vi "Move.vi"(8 "error in (no error)":errorcluster, 11 "Snake in":refnum<class "SnakeGame.lvclass">) -> (0 "error out":errorcluster, 3 "Snake out":refnum<class "SnakeGame.lvclass">)   [LabVIEW 2019, in "RT_Game.lvlib" / "SnakeGame.lvclass"]
uses:
  SnakeGame.lvclass
  SnakeGame.lvclass/SnakeGame.ctl
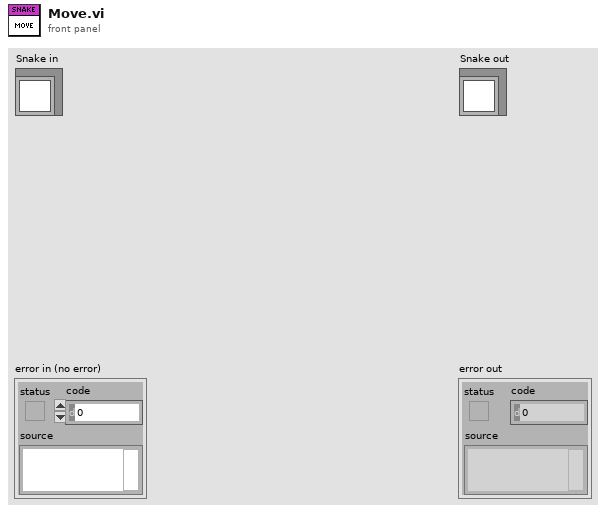
[diagram p1: front panel]
types:
  T1 = typedef "RT_Game.lvlib/SnakeGame.lvclass/Direction.ctl" = enum16{"Up", "Left", "Down", "Right"}
  T2 = typedef "RT_Game.lvlib/Game.lvclass/Coordinate.ctl" = cluster{"x":i16, "y":i16}
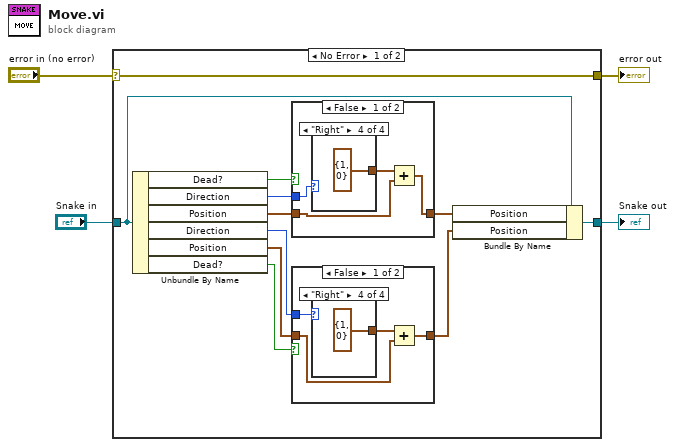
[diagram p0: block diagram]
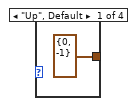
[diagram p2: hidden frame]
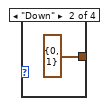
[diagram p3: hidden frame]
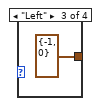
[diagram p4: hidden frame]
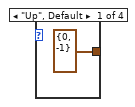
[diagram p6: hidden frame]
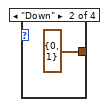
[diagram p7: hidden frame]
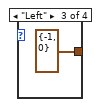
[diagram p8: hidden frame]
diagram:
  n1 = case shown="No Error" "error in (no error)" {
    selector: "error in (no error)" -> [w15 w35]
    tunnel: [w15 w35] -> w3
    tunnel: [w12 w34] -> w1
    tunnel: "Snake in" -> [w14 w34]
    frame No Error {
      n2 = Unbundle By Name(w14) -> ("Dead?"=w5:bool, "Direction"=w13:T1, "Position"=w11:T2, "Direction"=w8:T1, "Position"=w9:T2, "Dead?"=w6:bool)
      n3 = case shown="False" w5 {
        tunnel: w13 -> [w19 _]
        tunnel: w11 -> [w18 w24]
        tunnel: [w16 w24] -> w10
        frame False {
          n4 = case shown="\"Right\"" w19 {
            tunnel: [cluster{"x":i8, "y":i8} {"x"=0, "y"=-1} ("x") cluster{"x":i8, "y":i8} {"x"=0, "y"=1} ("x") cluster{"x":i8, "y":i8} {"x"=-1, "y"=0} ("x") cluster{"x":i8, "y":i8} {"x"=1, "y"=0} ("x")] -> w17
            frame "Up", Default {
            }
            frame "Down" {
            }
            frame "Left" {
            }
            frame "Right" {
            }
          }
          n5 = Add(x=w17, y=w18) -> (x+y=w16:T2)
        }
        frame True {
        }
      }
      n6 = case shown="False" w6 {
        tunnel: w9 -> [w27 w33]
        tunnel: w8 -> [w26 _]
        tunnel: [w25 w33] -> w7
        frame False {
          n7 = case shown="\"Right\"" w26 {
            tunnel: [cluster{"x":i8, "y":i8} {"x"=0, "y"=-1} ("x") cluster{"x":i8, "y":i8} {"x"=0, "y"=1} ("x") cluster{"x":i8, "y":i8} {"x"=-1, "y"=0} ("x") cluster{"x":i8, "y":i8} {"x"=1, "y"=0} ("x")] -> w28
            frame "Up", Default {
            }
            frame "Down" {
            }
            frame "Left" {
            }
            frame "Right" {
            }
          }
          n8 = Add(x=w28, y=w27) -> (x+y=w25:T2)
        }
        frame True {
        }
      }
      n9 = Bundle By Name(cluster=w14, "Position"=w10, "Position"=w7) -> (w12:refnum<class "SnakeGame.lvclass">)
    }
    frame Error {
    }
  }
  "error out" <- w3
  "Snake out" <- w1
